vi "Read Power Meter classes.vi"(11 "IMD in":refnum<class "IMD.lvclass">) -> (2 "Power Meter classes":refnum<class "Power Meter.lvclass">[](array[class]), 3 "IMD out":refnum<class "IMD.lvclass">)   [LabVIEW 2020, in "IMD.lvclass"]
uses:
  IMD.lvclass
  Instruments/Power Meter/Power Meter.lvclass
  IMD.lvclass/IMD.ctl
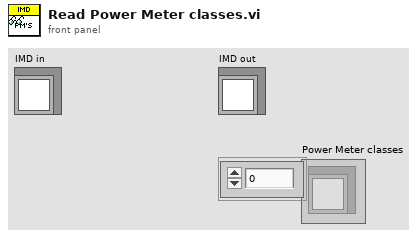
[diagram p1: front panel]
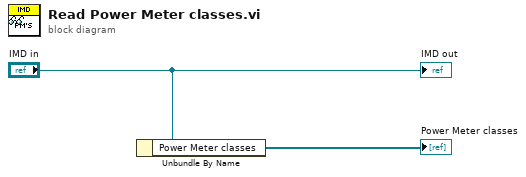
[diagram p0: block diagram]
diagram:
  n1 = Unbundle By Name("IMD in") -> ("Power Meter classes"=→"Power Meter classes":refnum<class "Power Meter.lvclass">[])
  "IMD out" <- "IMD in"
